vi "subAppendWfmArrays.vi"(1 "B":waveform(dbl)[](graph), 2 "A":waveform(dbl)[](graph)) -> (0 "Output":waveform(dbl)[](graph))   [LabVIEW 2017]
doc: "Appends <B>waveform B</B> to the end of <B>waveform A</B>. If the sampling rates do not match, the error cluster returns an error. The trigger time of <B>waveform B</B> is ignored."
uses:
  <vilib>/Waveform/WDTOps.llb/WDT Number of Waveform Samples DBL.vi
  <vilib>/Waveform/WDTOps.llb/WDT Append Waveforms DBL.vi
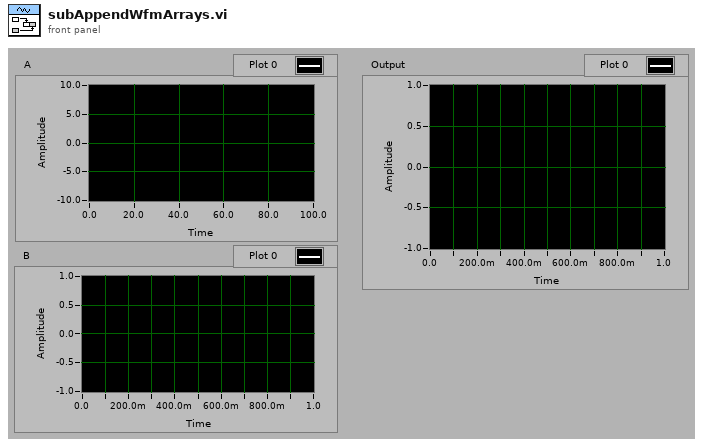
[diagram p1: front panel]
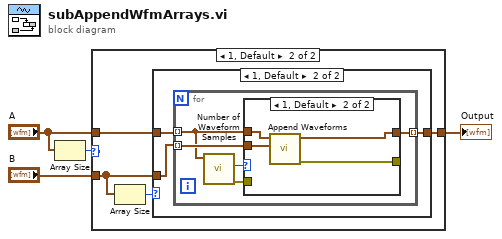
[diagram p0: block diagram]
diagram:
  n1 = Array Size(array="A") -> (size(s)=w2:i32)
  n2 = case shown="1, Default" w2 {
    tunnel: "A" -> [_ w9]
    tunnel: "B" -> [w5 w7]
    tunnel: [w5 w8] -> w3
    frame 0 {
      # "'A' waveform is empty"
    }
    frame 1, Default {
      n3 = Array Size(array=w7) -> (size(s)=w6:i32)
      n4 = case shown="1, Default" w6 {
        tunnel: w9 -> [w10 w13]
        tunnel: [w10 w12] -> w8
        tunnel: w7 -> [_ w11]
        frame 0 {
          # "'B' Waveform is empty."
        }
        frame 1, Default {
          n5 = for {
            tunnel: w13 -> [w16] mode=indexing
            tunnel: w11 -> [w17] mode=indexing
            tunnel: [w18] -> w12 mode=indexing
            n6 = call-poly <vilib>:"Number of Waveform Samples.vi"("waveform in"=w16) -> ("error out"=w14:errorcluster, "number of samples"=w15:i32)  [unwired: 8 in, 1 out]
            n7 = case shown="1, Default" w15 {
              tunnel: [w20 w24] -> w18
              tunnel: w17 -> [w20 w23]
              tunnel: w16 -> [_ w22]
              tunnel: [w19 w21] -> _
              tunnel: w14 -> [w19 _]
              frame 0 {
              }
              frame 1, Default {
                n8 = call-poly <vilib>:"Append Waveforms.vi"("waveform B"=w23, "waveform A"=w22) -> ("error out"=w21:errorcluster, "waveform out"=w24:waveform(dbl))  [unwired: 8 in]
              }
            }
          }
        }
      }
    }
  }
  "Output" <- w3
